vi "Parcial.vi"() -> ()   [LabVIEW 2017]
panel:
  in  "B4":bool
  in  "S3":bool
  in  "Modo":bool
  out "Ascensor":bool
  out "Subir1":bool
  out "Bajar2":bool
  out "Subir2":bool
  out "Bajar3":bool
  out "Subir3":bool
  out "Bajar4":bool
  in  "B3":bool
  in  "S2":bool
  in  "S1":bool
  in  "B2":bool
  in  "Cerrado":bool
  in  "Apertura":bool
  out "Piso":i8
  in  "4":bool
  in  "2":bool
  in  "3":bool
  in  "1":bool
  out "SP4":bool
  out "SP3":bool
  out "SP2":bool
  out "SP1":bool
  out "Flecha Arriba":bool
  out "Flecha Abajo":bool
  out "Numero4":bool
  out "Numero3":bool
  out "Numero2":bool
  out "Numero1":bool
  # "AUTOMÁTICO"
  # "MANUAL"
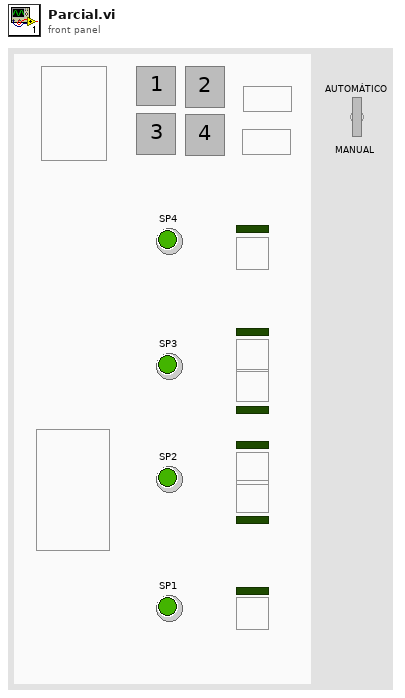
[diagram p1: front panel]
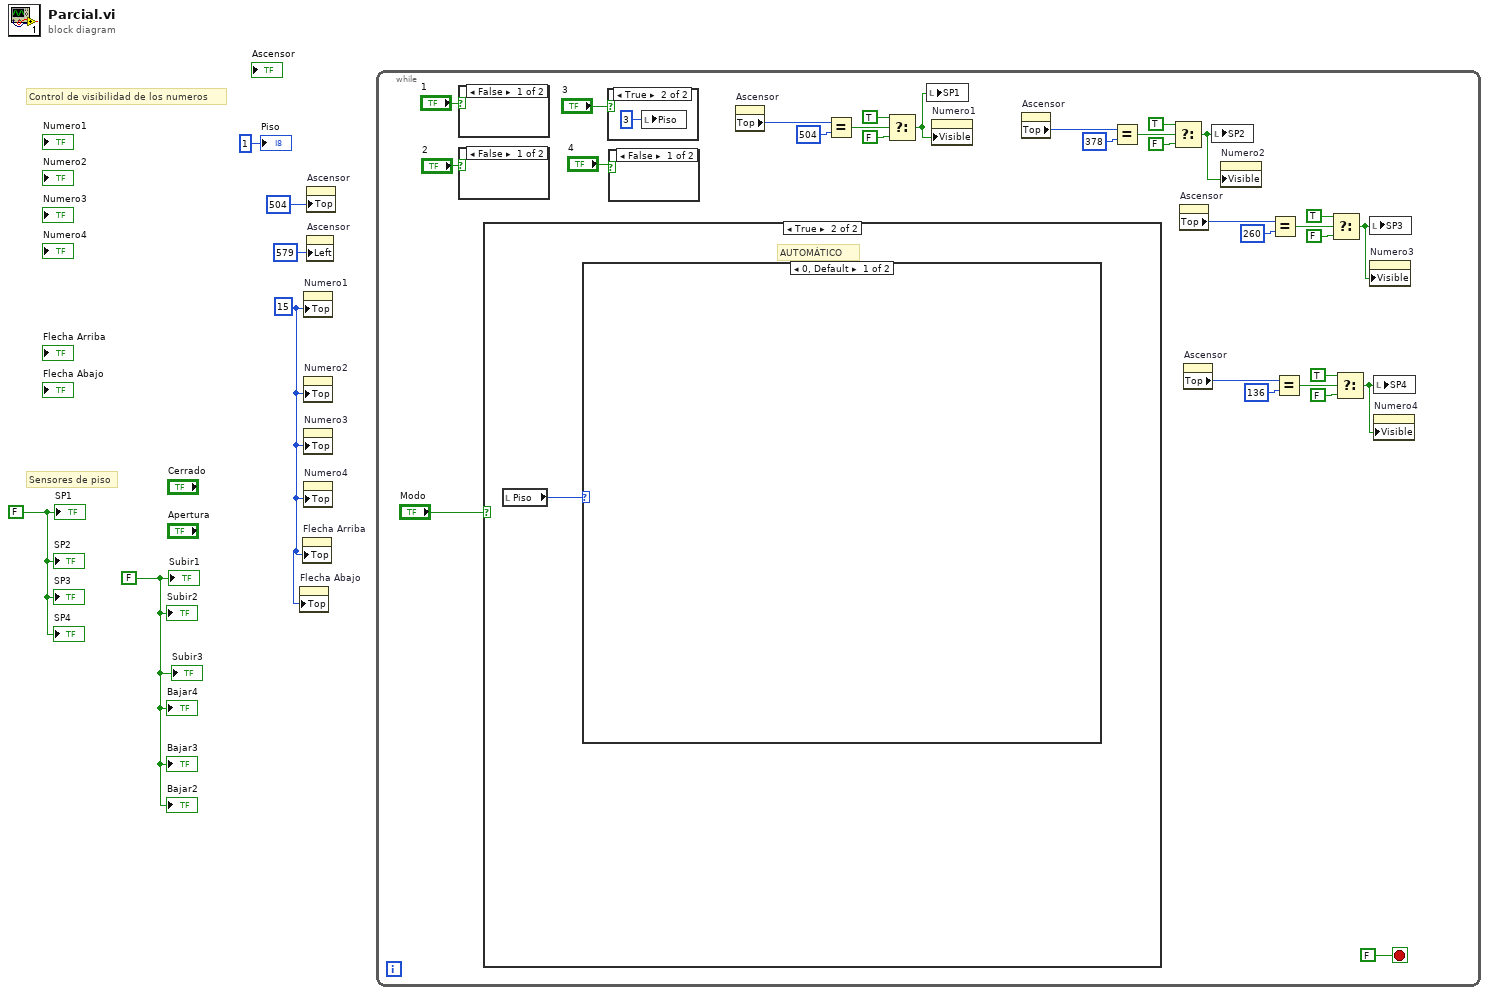
[diagram p0: block diagram]
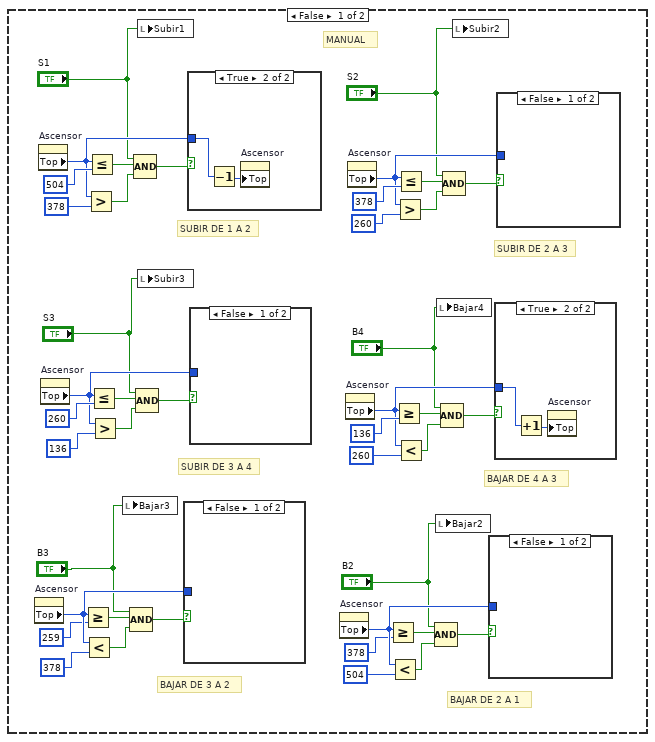
[diagram p2: hidden frame]
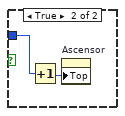
[diagram p3: hidden frame]
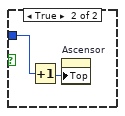
[diagram p4: hidden frame]
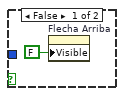
[diagram p5: hidden frame]
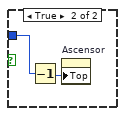
[diagram p6: hidden frame]
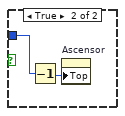
[diagram p7: hidden frame]
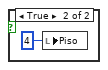
[diagram p10: hidden frame]
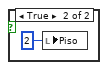
[diagram p12: hidden frame]
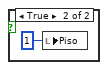
[diagram p13: hidden frame]
diagram:
  w2 = FALSE ("SP1")
  w3 = FALSE ("Subir1")
  w1 = 15 ("Position:Top")
  # "Sensores de piso"
  # "Control de visibilidad de los numeros"
  n1 = property on="Flecha Abajo" class="Bool (strict)"("Top"=w1) -> ()  [unwired: 2 in, 2 out]
  n2 = property on="Flecha Arriba" class="Bool (strict)"("Top"=w1) -> ()  [unwired: 2 in, 2 out]
  n3 = property on="Numero1" class="Bool (strict)"("Top"=w1) -> ()  [unwired: 2 in, 2 out]
  n4 = property on="Numero2" class="Bool (strict)"("Top"=w1) -> ()  [unwired: 2 in, 2 out]
  n5 = property on="Numero3" class="Bool (strict)"("Top"=w1) -> ()  [unwired: 2 in, 2 out]
  n6 = property on="Numero4" class="Bool (strict)"("Top"=w1) -> ()  [unwired: 2 in, 2 out]
  n7 = property on="Ascensor" class="Bool (strict)"("Top"=504 ("Position:Top")) -> ()  [unwired: 2 in, 2 out]
  n8 = property on="Ascensor" class="Bool (strict)"("Left"=579 ("Position:Left")) -> ()  [unwired: 2 in, 2 out]
  n9 = while {
    stop <- FALSE stop-if-true
    n10 = case shown="False" "1" {
      frame False {
      }
      frame True {
        n11 = local write "Piso"(i8 1 ("Piso")) -> ()
      }
    }
    n12 = case shown="False" "2" {
      frame False {
      }
      frame True {
        n13 = local write "Piso"(i8 2 ("Piso")) -> ()
      }
    }
    n14 = case shown="True" "Modo" {
      frame False {
        # "BAJAR DE 2 A 1"
        # "BAJAR DE 3 A 2"
        # "BAJAR DE 4 A 3"
        # "SUBIR DE 3 A 4"
        # "SUBIR DE 2 A 3"
        # "SUBIR DE 1 A 2"
        # "MANUAL"
        n15 = property on="Ascensor" class="Bool (strict)"() -> ("Top"=w52:i32)  [unwired: 2 in, 2 out]
        n16 = property on="Ascensor" class="Bool (strict)"() -> ("Top"=w59:i32)  [unwired: 2 in, 2 out]
        n17 = property on="Ascensor" class="Bool (strict)"() -> ("Top"=w57:i32)  [unwired: 2 in, 2 out]
        n18 = Greater Or Equal?(x=w52, y=259) -> (x >= y?=w44:bool)
        n19 = Less?(x=w52, y=378) -> (x < y?=w43:bool)
        n20 = Greater?(x=w59, y=378) -> (0:w78:bool)
        n21 = Less Or Equal?(x=w59, y=504) -> (x <= y?=w77:bool)
        n22 = Less Or Equal?(x=w57, y=260) -> (x <= y?=w67:bool)
        n23 = Greater?(x=w57, y=136) -> (0:w68:bool)
        n24 = local write "Bajar3"("B3") -> ()
        n25 = Compound Arithmetic op=AND("B3", w44, w43) -> (w45:bool)
        n26 = Compound Arithmetic op=AND("S1", w77, w78) -> (w76:bool)
        n27 = Compound Arithmetic op=AND("S3", w67, w68) -> (w66:bool)
        n28 = local write "Subir1"("S1") -> ()
        n29 = local write "Subir3"("S3") -> ()
        n30 = case shown="False" w45 {
          tunnel: w52 -> [_ w82]
          frame False {
          }
          frame True {
            n31 = Increment(x=w82) -> (x+1=w81:i32)
            n32 = property on="Ascensor" class="Bool (strict)"("Top"=w81) -> ()  [unwired: 2 in, 2 out]
          }
        }
        n33 = case shown="True" w76 {
          tunnel: w59 -> [_ w91]
          frame False {
          }
          frame True {
            n34 = Decrement(x=w91) -> (x-1=w90:i32)
            n35 = property on="Ascensor" class="Bool (strict)"("Top"=w90) -> ()  [unwired: 2 in, 2 out]
          }
        }
        n36 = case shown="False" w66 {
          tunnel: w57 -> [_ w87]
          frame False {
          }
          frame True {
            n37 = Decrement(x=w87) -> (x-1=w86:i32)
            n38 = property on="Ascensor" class="Bool (strict)"("Top"=w86) -> ()  [unwired: 2 in, 2 out]
          }
        }
        n39 = property on="Ascensor" class="Bool (strict)"() -> ("Top"=w53:i32)  [unwired: 2 in, 2 out]
        n40 = property on="Ascensor" class="Bool (strict)"() -> ("Top"=w56:i32)  [unwired: 2 in, 2 out]
        n41 = property on="Ascensor" class="Bool (strict)"() -> ("Top"=w58:i32)  [unwired: 2 in, 2 out]
        n42 = Greater Or Equal?(x=w53, y=378) -> (x >= y?=w48:bool)
        n43 = Less?(x=w53, y=504) -> (x < y?=w51:bool)
        n44 = Greater Or Equal?(x=w56, y=136) -> (x >= y?=w63:bool)
        n45 = Greater?(x=w58, y=260) -> (0:w73:bool)
        n46 = Less Or Equal?(x=w58, y=378) -> (x <= y?=w72:bool)
        n47 = Less?(x=w56, y=260) -> (x < y?=w60:bool)
        n48 = Compound Arithmetic op=AND("B2", w48, w51) -> (w49:bool)
        n49 = local write "Bajar2"("B2") -> ()
        n50 = local write "Bajar4"("B4") -> ()
        n51 = Compound Arithmetic op=AND("B4", w63, w60) -> (w62:bool)
        n52 = Compound Arithmetic op=AND("S2", w72, w73) -> (w71:bool)
        n53 = local write "Subir2"("S2") -> ()
        n54 = case shown="False" w49 {
          tunnel: w53 -> [_ w80]
          frame False {
          }
          frame True {
            n55 = Increment(x=w80) -> (x+1=w79:i32)
            n56 = property on="Ascensor" class="Bool (strict)"("Top"=w79) -> ()  [unwired: 2 in, 2 out]
          }
        }
        n57 = case shown="True" w62 {
          tunnel: w56 -> [_ w85]
          frame False {
            n58 = property on="Flecha Arriba" class="Bool (strict)"("Visible"=FALSE) -> ()  [unwired: 2 in, 2 out]
          }
          frame True {
            n59 = Increment(x=w85) -> (x+1=w84:i32)
            n60 = property on="Ascensor" class="Bool (strict)"("Top"=w84) -> ()  [unwired: 2 in, 2 out]
          }
        }
        n61 = case shown="False" w71 {
          tunnel: w58 -> [_ w89]
          frame False {
          }
          frame True {
            n62 = Decrement(x=w89) -> (x-1=w88:i32)
            n63 = property on="Ascensor" class="Bool (strict)"("Top"=w88) -> ()  [unwired: 2 in, 2 out]
          }
        }
      }
      frame True {
        # "AUTOMÁTICO"
        n64 = local read "Piso"() -> (w92:i8)
        n65 = case shown="0, Default" w92 {
          frame 0, Default {
          }
          frame 1 {
          }
        }
      }
    }
    n66 = case shown="True" "3" {
      frame False {
      }
      frame True {
        n67 = local write "Piso"(i8 3 ("Piso")) -> ()
      }
    }
    n68 = case shown="False" "4" {
      frame False {
      }
      frame True {
        n69 = local write "Piso"(i8 4 ("Piso")) -> ()
      }
    }
    n70 = property on="Ascensor" class="Bool (strict)"() -> ("Top"=w27:i32)  [unwired: 2 in, 2 out]
    n71 = Equal?(x=w27, y=504) -> (x = y?=w30:bool)
    n72 = Select(t=TRUE, s=w30, f=FALSE) -> (s? t:f=w7:bool)
    n73 = local write "SP1"(w7) -> ()
    n74 = property on="Numero1" class="Bool (strict)"("Visible"=w7) -> ()  [unwired: 2 in, 2 out]
    n75 = property on="Ascensor" class="Bool (strict)"() -> ("Top"=w24:i32)  [unwired: 2 in, 2 out]
    n76 = Equal?(x=w24, y=378) -> (x = y?=w21:bool)
    n77 = Select(t=TRUE, s=w21, f=FALSE) -> (s? t:f=w10:bool)
    n78 = property on="Ascensor" class="Bool (strict)"() -> ("Top"=w14:i32)  [unwired: 2 in, 2 out]
    n79 = property on="Ascensor" class="Bool (strict)"() -> ("Top"=w17:i32)  [unwired: 2 in, 2 out]
    n80 = local write "SP2"(w10) -> ()
    n81 = property on="Numero2" class="Bool (strict)"("Visible"=w10) -> ()  [unwired: 2 in, 2 out]
    n82 = Equal?(x=w14, y=260) -> (x = y?=w11:bool)
    n83 = Equal?(x=w17, y=136) -> (x = y?=w20:bool)
    n84 = Select(t=TRUE, s=w11, f=FALSE) -> (s? t:f=w9:bool)
    n85 = Select(t=TRUE, s=w20, f=FALSE) -> (s? t:f=w8:bool)
    n86 = local write "SP3"(w9) -> ()
    n87 = property on="Numero3" class="Bool (strict)"("Visible"=w9) -> ()  [unwired: 2 in, 2 out]
    n88 = local write "SP4"(w8) -> ()
    n89 = property on="Numero4" class="Bool (strict)"("Visible"=w8) -> ()  [unwired: 2 in, 2 out]
  }
  "SP2" <- w2
  "SP3" <- w2
  "SP4" <- w2
  "Piso" <- i8 1 ("Piso")
  "Bajar4" <- w3
  "Subir3" <- w3
  "Bajar3" <- w3
  "Subir2" <- w3
  "Bajar2" <- w3
  "Subir1" <- w3
  "SP1" <- w2
